vi "Prompt for Step--Update State Data.vi"(8 "error in (no error)":errorcluster, 9 "Data":variant, 10 "Argument":string, 11 "Mouse Action in":refnum<class "Mouse Action.lvclass">) -> (0 "error out":errorcluster, 3 "Mouse Action out":refnum<class "Mouse Action.lvclass">)   [LabVIEW 2020, in "MacroAssert.lvlib" / "Mouse Action.lvclass"]
doc: "Updates the state data within the \"Prompt for Step\" VI."
uses:
  Mouse Action.lvclass
  Mouse Action Type.ctl
  Button.ctl
  Click Type.ctl
  Relative Movement Type.ctl
  Action Step/Action Step.lvclass
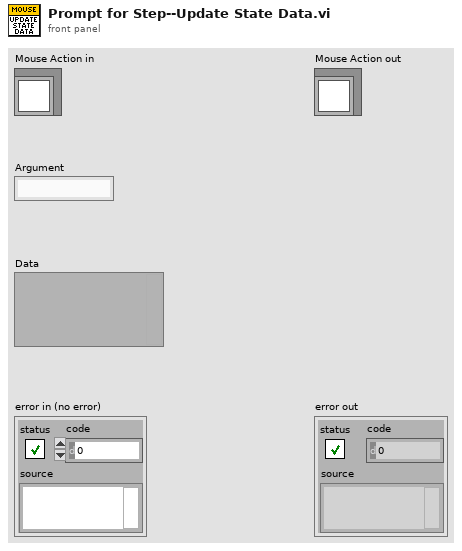
[diagram p1: front panel]
types:
  T1 = typedef "MacroAssert.lvlib/Mouse Action.lvclass/Mouse Action Type.ctl" = enum16{"Click", "Absolute Move", "Absolute Move and Click", "Relative Move", "Relative Move and Click", "Wheel Up", "Wheel Down"}
  T2 = typedef "MacroAssert.lvlib/Mouse Action.lvclass/Button.ctl" = enum16{"Left", "Right", "Middle"}
  T3 = typedef "MacroAssert.lvlib/Mouse Action.lvclass/Click Type.ctl" = enum16{"Normal", "Hold", "Release"}
  T4 = typedef "MacroAssert.lvlib/Mouse Action.lvclass/Relative Movement Type.ctl" = enum16{"Pixels from Current Position", "Pixels from Top-Left of Control", "Pixels from Top-Left of Window", "Percentage from Top-Left of Control", "Percentage from Top-Left of Window", "Percentage from Top-Left of Screen"}
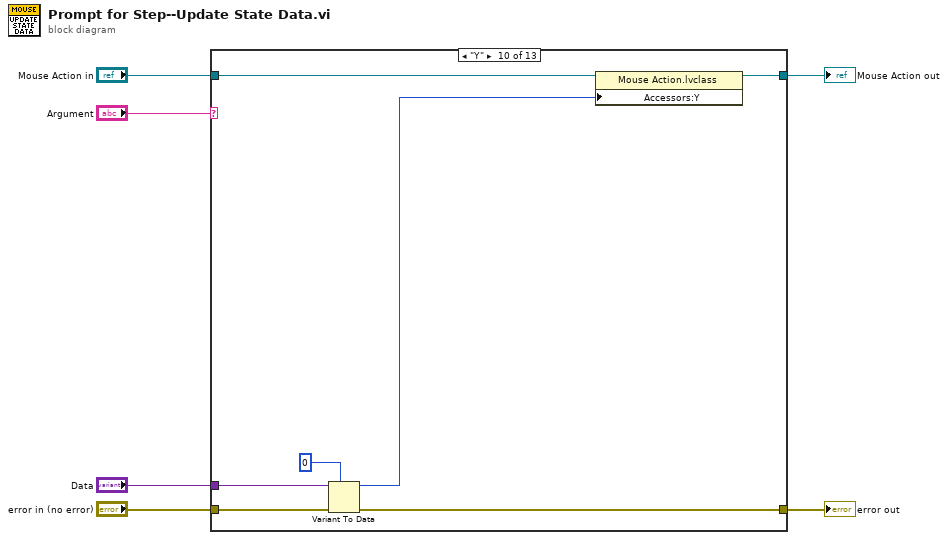
[diagram p0: block diagram]
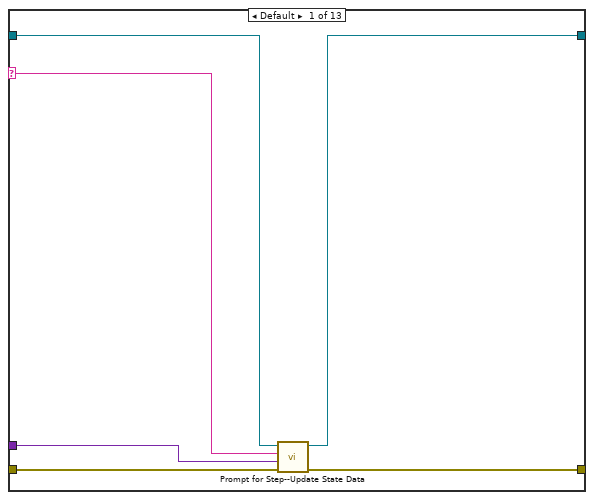
[diagram p2: hidden frame]
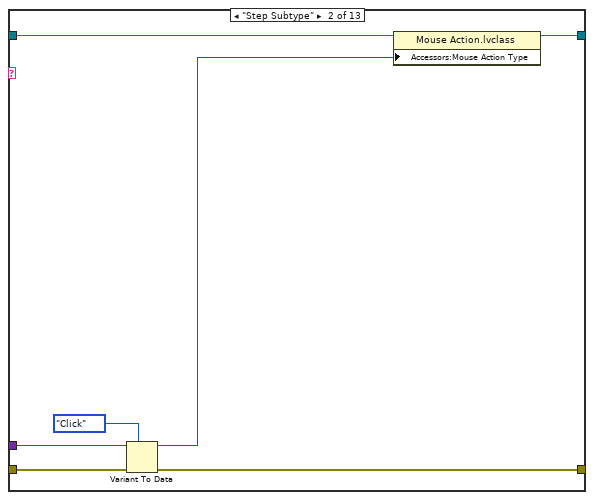
[diagram p3: hidden frame]
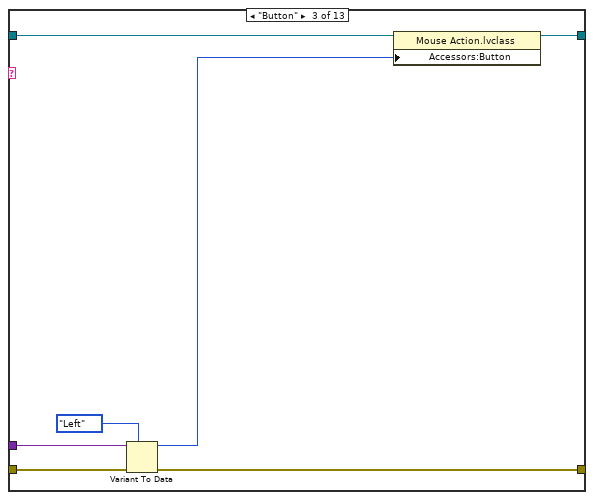
[diagram p4: hidden frame]
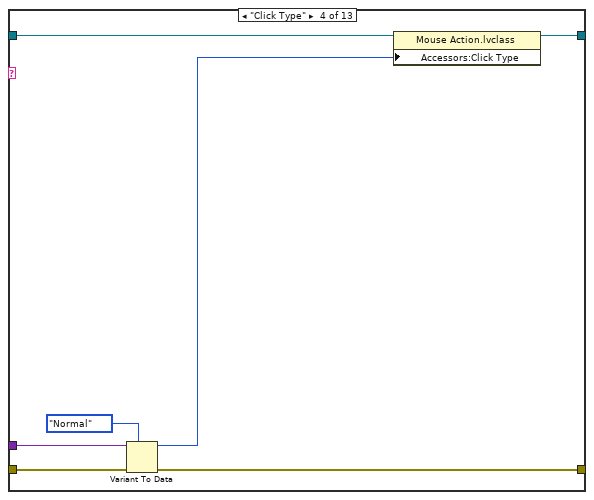
[diagram p5: hidden frame]
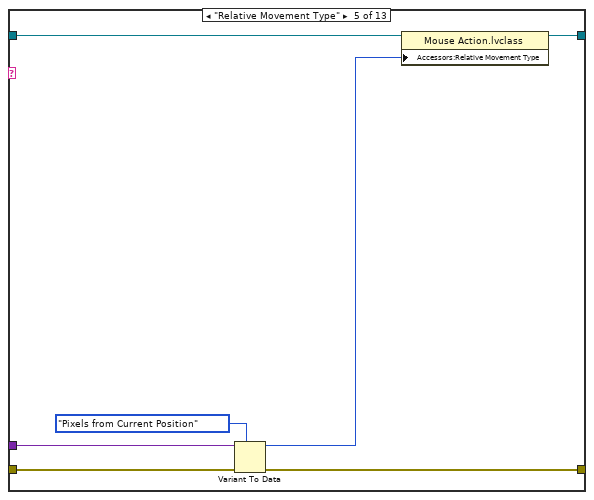
[diagram p6: hidden frame]
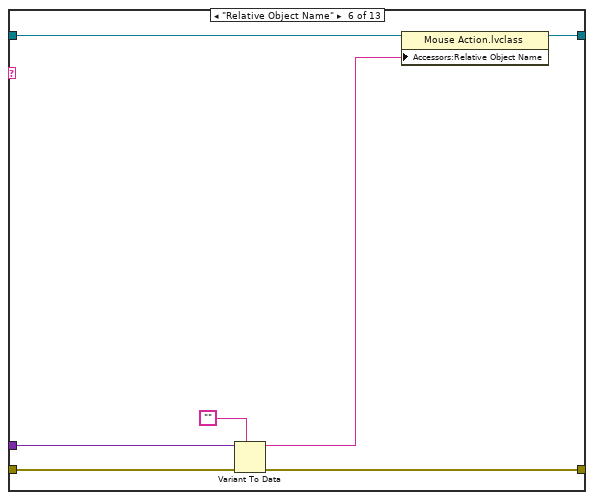
[diagram p7: hidden frame]
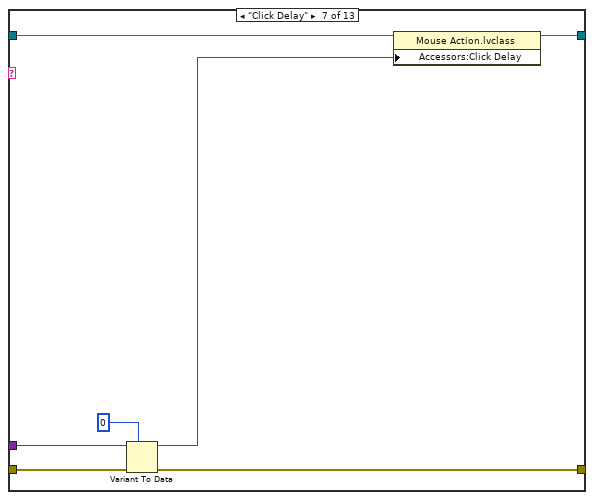
[diagram p8: hidden frame]
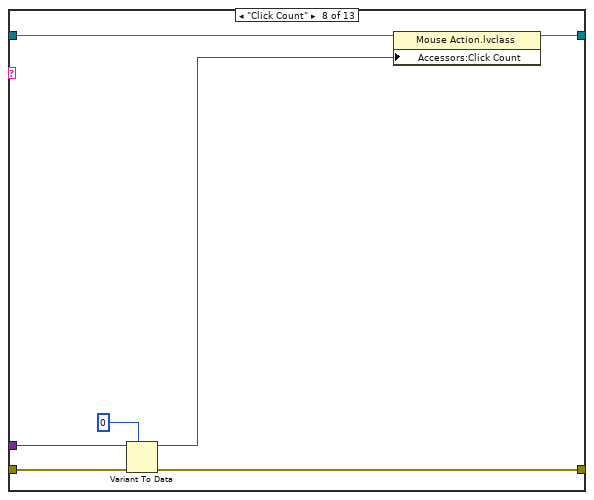
[diagram p9: hidden frame]
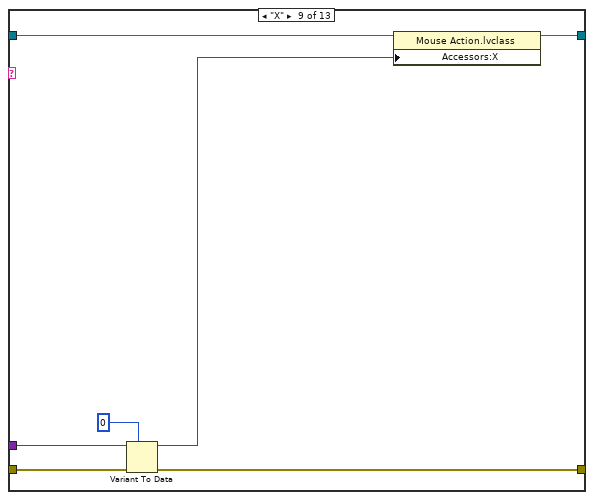
[diagram p10: hidden frame]
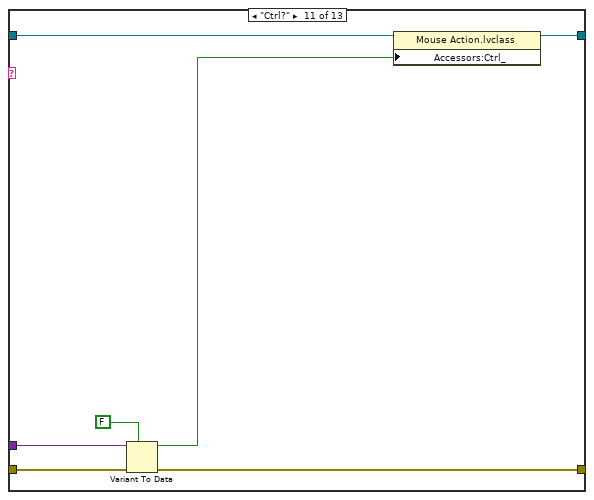
[diagram p11: hidden frame]
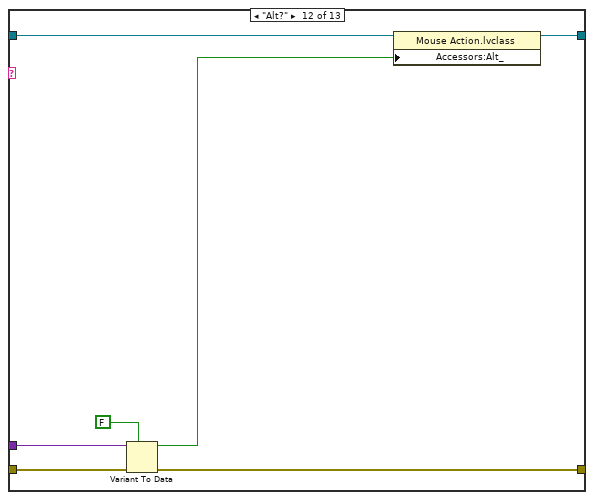
[diagram p12: hidden frame]
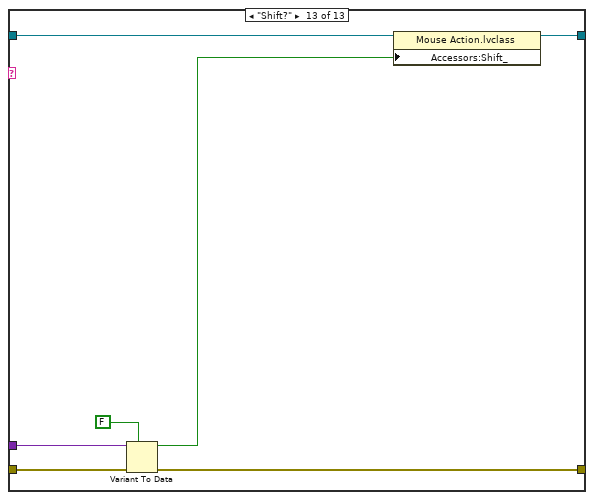
[diagram p13: hidden frame]
diagram:
  n1 = case shown="\"Y\"" "Argument" {
    selector: "Argument" -> [w9 _ _ _ _ _ _ _ _ _ _ _ _]
    tunnel: "Mouse Action in" -> [w8 w19 w26 w33 w36 w44 w54 w61 w68 w75 w82 w89 w96]
    tunnel: "error in (no error)" -> [w12 w17 w24 w31 w40 w47 w52 w59 w66 w73 w80 w87 w94]
    tunnel: [w7 w18 w25 w32 w34 w42 w53 w60 w67 w74 w81 w88 w95] -> w2
    tunnel: [w11 w16 w23 w30 w39 w46 w51 w58 w65 w72 w79 w86 w93] -> w1
    tunnel: "Data" -> [w10 w14 w21 w28 w37 w45 w50 w57 w64 w71 w78 w85 w92]
    frame Default {
      n2 = call-parent "Prompt for Step--Update State Data.vi"("error in (no error)"=w12, "Data"=w10, "Argument"=w9, "Step in"=w8) -> ("error out"=w11:errorcluster, "Step out"=w7:refnum<class "Mouse Action.lvclass">)  [unwired: 6 in]
    }
    frame "Step Subtype" {
      n3 = Variant To Data(error in=w17, type=Mouse_Action_Type."Click" ("Mouse Action Type"), Variant=w14) -> (data=w13:T1, error out=w16:errorcluster)
      n4 = property class="Mouse Action.lvclass"(reference=w19, "Accessors:Mouse Action Type"=w13) -> (reference out=w18:refnum<class "Mouse Action.lvclass">)  [unwired: 1 in, 1 out]
    }
    frame "Button" {
      n5 = Variant To Data(error in=w24, type=Button."Left" ("Button"), Variant=w21) -> (data=w20:T2, error out=w23:errorcluster)
      n6 = property class="Mouse Action.lvclass"(reference=w26, "Accessors:Button"=w20) -> (reference out=w25:refnum<class "Mouse Action.lvclass">)  [unwired: 1 in, 1 out]
    }
    frame "Click Type" {
      n7 = Variant To Data(error in=w31, type=Click_Type."Normal" ("Click Type"), Variant=w28) -> (data=w27:T3, error out=w30:errorcluster)
      n8 = property class="Mouse Action.lvclass"(reference=w33, "Accessors:Click Type"=w27) -> (reference out=w32:refnum<class "Mouse Action.lvclass">)  [unwired: 1 in, 1 out]
    }
    frame "Relative Movement Type" {
      n9 = Variant To Data(error in=w40, type=Relative_Movement_Type."Pixels from Current Position" ("Relative Movement Type"), Variant=w37) -> (data=w35:T4, error out=w39:errorcluster)
      n10 = property class="Mouse Action.lvclass"(reference=w36, "Accessors:Relative Movement Type"=w35) -> (reference out=w34:refnum<class "Mouse Action.lvclass">)  [unwired: 1 in, 1 out]
    }
    frame "Relative Object Name" {
      n11 = Variant To Data(error in=w47, type="", Variant=w45) -> (data=w43:string, error out=w46:errorcluster)
      n12 = property class="Mouse Action.lvclass"(reference=w44, "Accessors:Relative Object Name"=w43) -> (reference out=w42:refnum<class "Mouse Action.lvclass">)  [unwired: 1 in, 1 out]
    }
    frame "Click Delay" {
      n13 = Variant To Data(error in=w52, type=0, Variant=w50) -> (data=w49:i32, error out=w51:errorcluster)
      n14 = property class="Mouse Action.lvclass"(reference=w54, "Accessors:Click Delay"=w49) -> (reference out=w53:refnum<class "Mouse Action.lvclass">)  [unwired: 1 in, 1 out]
    }
    frame "Click Count" {
      n15 = Variant To Data(error in=w59, type=0, Variant=w57) -> (data=w56:i32, error out=w58:errorcluster)
      n16 = property class="Mouse Action.lvclass"(reference=w61, "Accessors:Click Count"=w56) -> (reference out=w60:refnum<class "Mouse Action.lvclass">)  [unwired: 1 in, 1 out]
    }
    frame "X" {
      n17 = Variant To Data(error in=w66, type=0, Variant=w64) -> (data=w63:i32, error out=w65:errorcluster)
      n18 = property class="Mouse Action.lvclass"(reference=w68, "Accessors:X"=w63) -> (reference out=w67:refnum<class "Mouse Action.lvclass">)  [unwired: 1 in, 1 out]
    }
    frame "Y" {
      n19 = Variant To Data(error in=w73, type=0, Variant=w71) -> (data=w70:i32, error out=w72:errorcluster)
      n20 = property class="Mouse Action.lvclass"(reference=w75, "Accessors:Y"=w70) -> (reference out=w74:refnum<class "Mouse Action.lvclass">)  [unwired: 1 in, 1 out]
    }
    frame "Ctrl?" {
      n21 = Variant To Data(error in=w80, type=FALSE, Variant=w78) -> (data=w77:bool, error out=w79:errorcluster)
      n22 = property class="Mouse Action.lvclass"(reference=w82, "Accessors:Ctrl_"=w77) -> (reference out=w81:refnum<class "Mouse Action.lvclass">)  [unwired: 1 in, 1 out]
    }
    frame "Alt?" {
      n23 = Variant To Data(error in=w87, type=FALSE, Variant=w85) -> (data=w84:bool, error out=w86:errorcluster)
      n24 = property class="Mouse Action.lvclass"(reference=w89, "Accessors:Alt_"=w84) -> (reference out=w88:refnum<class "Mouse Action.lvclass">)  [unwired: 1 in, 1 out]
    }
    frame "Shift?" {
      n25 = Variant To Data(error in=w94, type=FALSE, Variant=w92) -> (data=w91:bool, error out=w93:errorcluster)
      n26 = property class="Mouse Action.lvclass"(reference=w96, "Accessors:Shift_"=w91) -> (reference out=w95:refnum<class "Mouse Action.lvclass">)  [unwired: 1 in, 1 out]
    }
  }
  "error out" <- w1
  "Mouse Action out" <- w2
